vi "PXI-2510 RT Driver VI.vi"(6 "Device Clock":string, 9 "Device Inputs FIFO":refnum<k33>, 11 "Device Reference":T1 format="%.0x") -> ()   [LabVIEW 2011, in "PXI-2510 Custom Device.lvlib"]
uses:
  PXI-2510 Custom Device.lvlib
  <vilib>/NI Veristand/Custom Device API/Custom Device Item Ref.ctl
  <vilib>/NI Veristand/Custom Device API/Custom Device Channel Type.ctl
  <vilib>/Platform/TimedLoop/XDataNode/timing_clust.ctl
  <vilib>/Platform/TimedLoop/XDataNode/nitl_modes.ctl
  <vilib>/Platform/TimedLoop/XDataNode/wakeup.ctl
  <vilib>/NI Veristand/Custom Device API/Get Item Property (String).vi
  FIU Global Strings.vi
  <vilib>/Platform/TimedLoop/XDataNode/XDataNode.xnode
  <vilib>/Platform/TimedLoop/XDataNode/XDNodeRunTimeDep.lvlib
  <vilib>/NI Veristand/Custom Device API/Custom Device API.lvlib
panel:
  in  "Status Notifier":refnum<notifier>
  # "Custom Device Template\nv1.0"
  # "Use this template as a starting point for creating a custom device code module. The input controls shown here are specially named controls that the system will use to provide the device loop with data. The controls are not required for the device loop to run. For instance, if the device doesn't produce any output data, then you don't need the Device Outputs FIFO control. If you do use these controls, however, they need to have these exact names to be functional."
  # "The optional status notifier element is used to notify the RT engine of the last state of the custom device, and to indicate the device has completed execution. If this control is not used, a default No Error value is returned to the system when the device finishes execution."
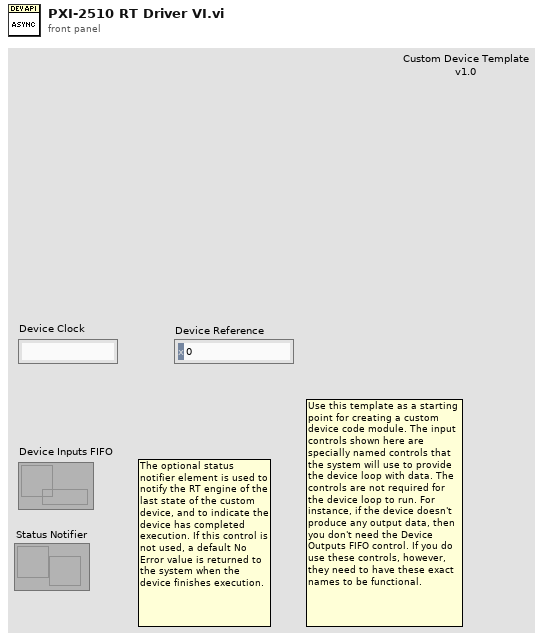
[diagram p1: front panel]
types:
  T1 = typedef "Custom Device API.lvlib/Custom Device Item Ref.ctl" = u64
  T2 = typedef "Custom Device API.lvlib/Custom Device Channel Type.ctl" = enum16{"Input", "Output"}
  T3 = typedef "Custom Device API.lvlib/Custom Device Timed Loop Priority.ctl" = enum32{"Low", "Medium", "High"}
  T4 = typedef "XDNodeRunTimeDep.lvlib/timing_clust.ctl" = cluster{"Expected End [f-1]":u64, "Actual End [f-1]":u64, "Finished Late? [f-1]":bool, "Expected End [i-1]":u64, "Actual End [i-1]":u64, "Finished Late? [i-1]":bool, "Expected Start [i]":u64, "Actual Start [i]":u64, "Expected Start [f]":u64, "Actual Start [f]":u64, "Source Name":string, "Structure Name":string, "Period":i64, "Deadline":i64, "Offset":i64, "Start":i64, "Priority":i32, "Timeout":i32, "Mode":T5, "Wakeup Reason":T6, "Error":errorcluster, "Source Type":string, "Secondary Source Type":string, "Global End Time":u64, "Global Start Time":u64, "Frame Duration":u64, "Iteration Duration":u64, "Assigned CPU":i32, "I/O Scan Engine Mode":u32}
  T5 = typedef "XDNodeRunTimeDep.lvlib/nitl_modes.ctl" = enum32{"No Change", "Process missed periods, maintain original phase", "Discard missed periods, maintain original phase", "Process missed periods, ignore original phase", "Discard missed periods, ignore original phase"}
  T6 = typedef "XDNodeRunTimeDep.lvlib/wakeup.ctl" = enum32{"Normal", "Aborted", "Asynchronous wakeup", "Timing source error", "Timed loop error", "Timeout"}
  T7 = enum16{"Default", "Fault A0 to FB A", "Fault A1 to FB A", "Fault A2 to FB A", "Fault A3 to FB A", "Fault Bus A Open"}
  T8 = enum16{"Default", "Fault B0 to FB B", "Fault B1 to FB B", "Fault B2 to FB B", "Fault B3 to FB B", "Fault Bus B Open"}
  T9 = enum16{"Default", "DUT Pass Through", "DUT Open", "DUT Pass Through and FB A", "DUT Pass Through and FB B", "DUT FB A", "DUT FB B"}
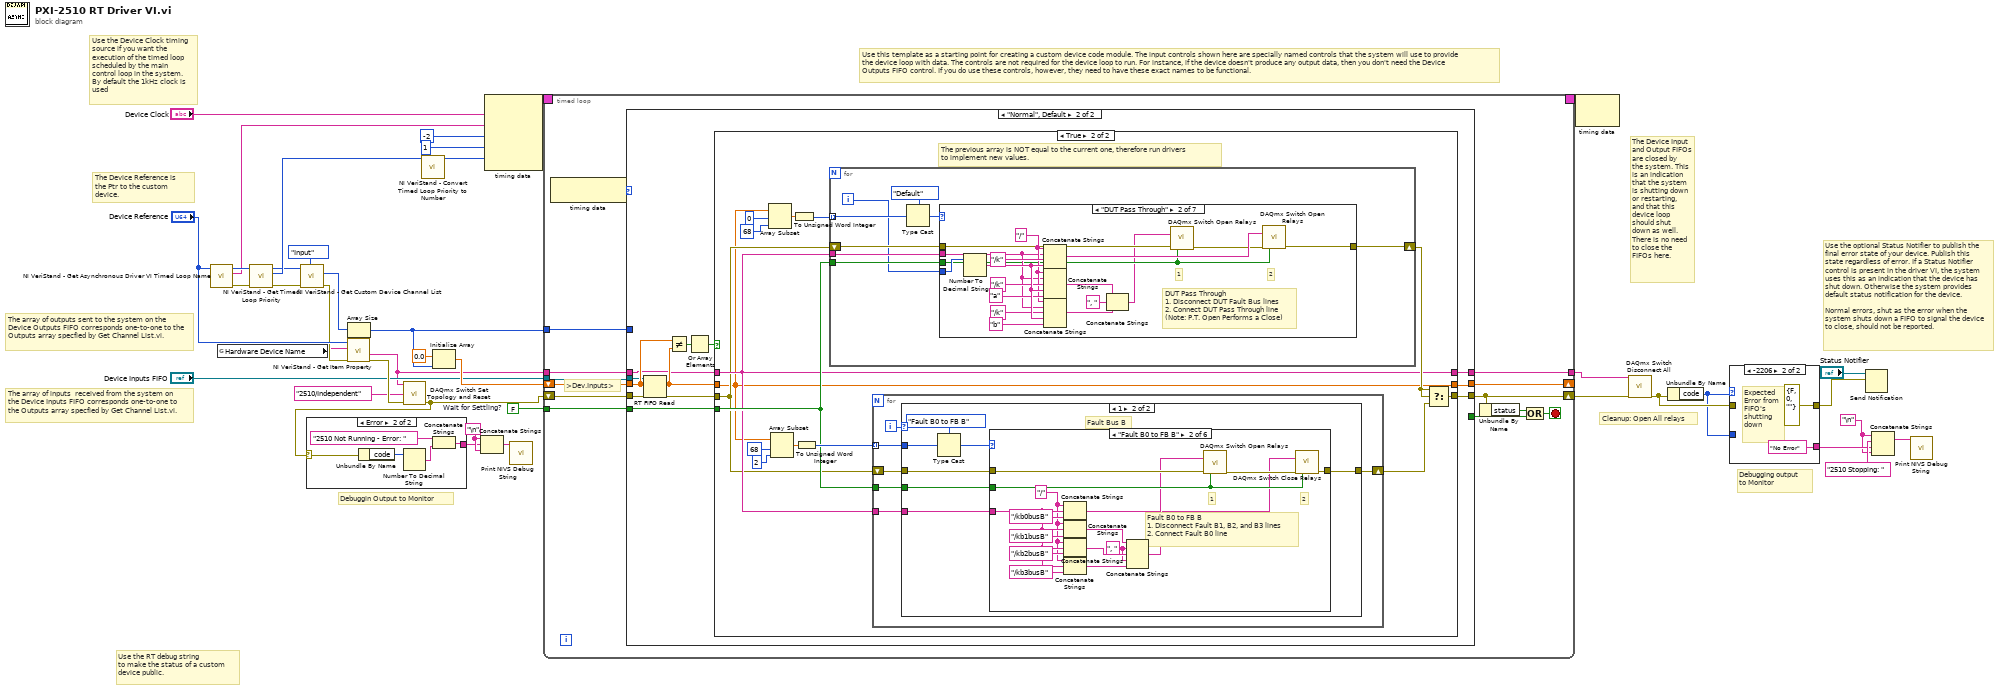
[diagram p0: block diagram]
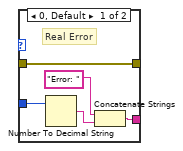
[diagram p2: hidden frame]
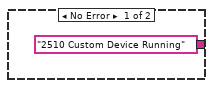
[diagram p3: hidden frame]
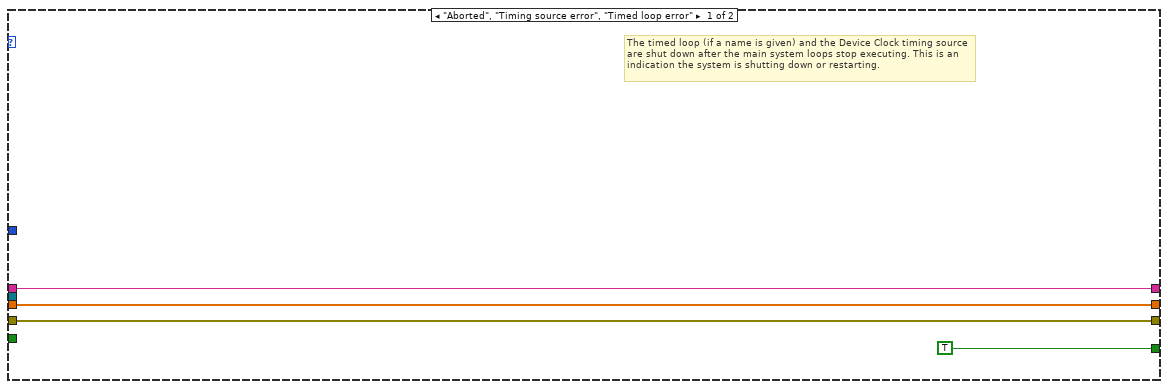
[diagram p4: hidden frame]
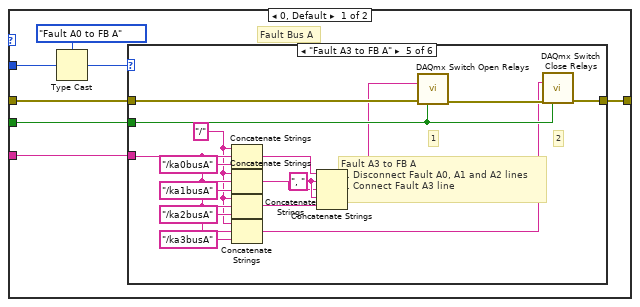
[diagram p6: hidden frame]
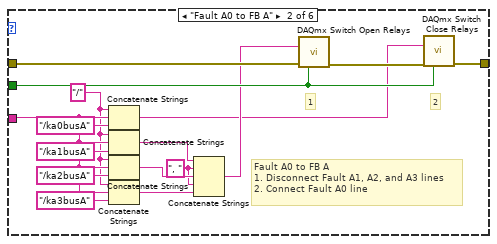
[diagram p8: hidden frame]
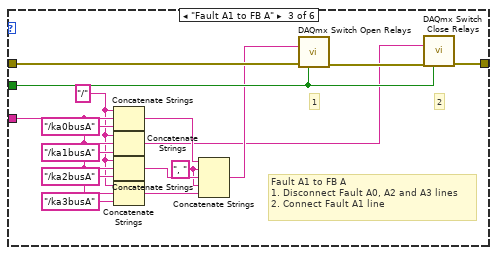
[diagram p9: hidden frame]
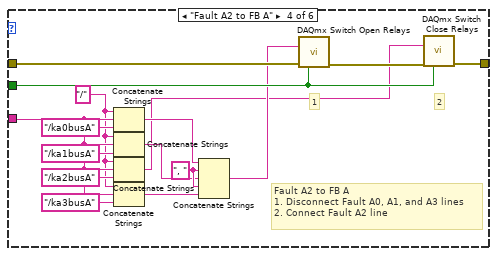
[diagram p10: hidden frame]
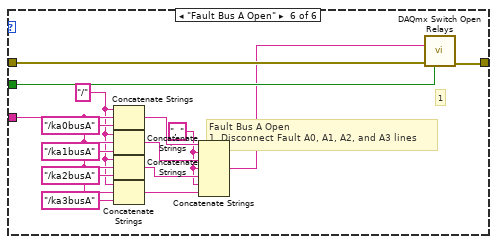
[diagram p11: hidden frame]
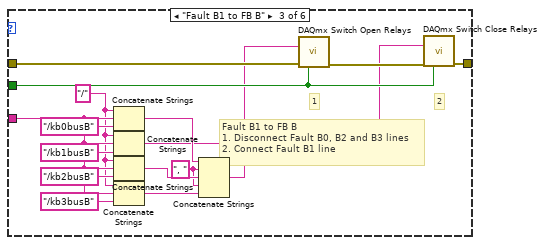
[diagram p13: hidden frame]
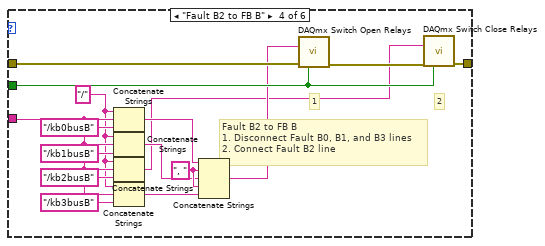
[diagram p14: hidden frame]
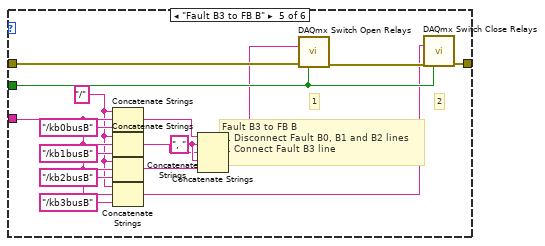
[diagram p15: hidden frame]
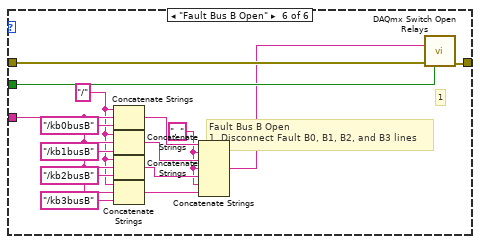
[diagram p16: hidden frame]
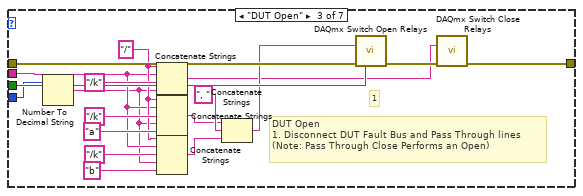
[diagram p18: hidden frame]
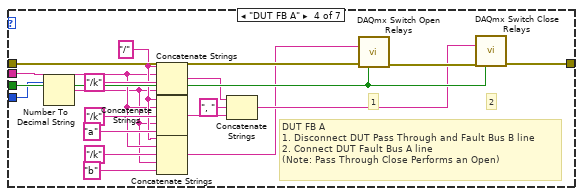
[diagram p19: hidden frame]
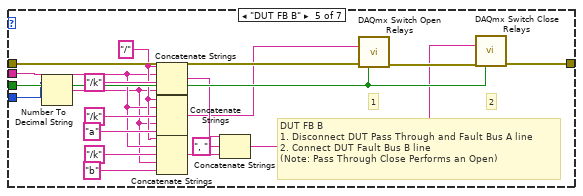
[diagram p20: hidden frame]
diagram:
  w4 = "\n"
  w14 = "\n"
  w24 = FALSE  # Wait for Settling?
  # "Debugging output\nto Monitor"
  # "Debuggin Output to Monitor"
  # "Cleanup: Open All relays"
  # "The array of inputs  received from the system on the Device Inputs FIFO corresponds one-to-one to the Outputs array specfied by Get Channel List.vi."
  # "Use the optional Status Notifier to publish the final error state of your device. Publish this state regardless of error. If a Status Notifier control is present in the driver VI, the system uses this as an indication that the device has shut down. Otherwise the system provides default status notification for the device.\n\nNormal errors, shut as the error when the system shuts down a FIFO to signal the device to close, should not be reported."
  # "Use the RT debug string\nto make the status of a custom\ndevice public."
  # "The Device Input and Output FIFOs are closed by the system. This is an indication that the system is shutting down or restarting, and that this device loop should shut down as well. There is no need to close the FIFOs here."
  # "The array of outputs sent to the system on the Device Outputs FIFO corresponds one-to-one to the Outputs array specfied by Get Channel List.vi."
  # "The Device Reference is\nthe Ptr to the custom device."
  # "Use the Device Clock timing source if you want the execution of the timed loop scheduled by the main control loop in the system. \nBy default the 1kHz clock is used"
  # "Use this template as a starting point for creating a custom device code module. The input controls shown here are specially named controls that the system will use to provide the device loop with data. The controls are not required for the device loop to run. For instance, if the device doesn't produce any output data, then you don't need the Device Outputs FIFO control. If you do use these controls, however, they need to have these exact names to be functional."
  n1 = call <vilib>:"NI VeriStand - Get Asynchronous Driver VI Timed Loop Name.vi"("Device Ref in"="Device Reference") -> ("error out"=w31:errorcluster, "Device Timed Loop Name"=w34:string, "Device Ref out"=w39:T1)  [unwired: 1 in, 7 out]
  n2 = global read "FIU Global Strings.vi" "Hardware Device Name"() -> (w19:string)
  n3 = call <vilib>:"NI VeriStand - Get Timed Loop Priority.vi"("error in (no error)"=w31, "Device Ref in"=w39) -> ("error out"=w16:errorcluster, "Priority"=w29:T3, "Device Ref out"=w17:T1)  [unwired: 7 out]
  n4 = call <vilib>:"NI VeriStand - Get Custom Device Channel List.vi"("Channel Type"=Custom_Device_Channel_Type."Input", "error in (no error)"=w16, "Device Ref in"=w17) -> ("error out"=w20:errorcluster, "Specified Channel Ref List"=w30:T1[])  [unwired: 7 out]
  n5 = call-poly <vilib>:"NI VeriStand - Get Item Property.vi"("error in (no error)"=w20, "Property Name"=w19, "Item Ref in"="Device Reference") -> ("error out"=w18:errorcluster, "Value"=w2:string)  [unwired: 5 in, 2 out]
  n6 = Array Size(array=w30) -> (size(s)=w25:i32)
  n7 = call <vilib>:"DAQmx Switch Set Topology and Reset.vi"("switch device"=w2, "topology name"="2510/Independent" ("string"), "error in"=w18) -> ("error out"=w1:errorcluster)  [unwired: 12 out]
  n8 = case shown="Error" w1 {
    selector: w1 -> [_ w41]
    tunnel: ["2510 Custom Device Running" ("String to write") w42] -> w13
    frame No Error {
    }
    frame Error {
      n9 = Unbundle By Name(w41) -> ("code"=w45:i32)
      n10 = Number To Decimal String(number=w45) -> (decimal integer string=w43:string)  [unwired: 1 in]
      n11 = Concatenate Strings("2510 Not Running - Error: " ("String to write"), w43) -> (w42:string)
    }
  }
  n12 = call <vilib>:"NI VeriStand - Convert Timed Loop Priority to Number.vi"("Priority"=w29) -> ("Numeric Priority"=w28:i32)  [unwired: 10 out]
  n13 = Initialize Array(0.0 ("element"), w25) -> (w35:dbl[])
  n14 = Concatenate Strings(w14, w13, w14) -> (w12:string)
  n15 = node-c288("Device Clock", w34, -2 ("Processor"), i64 1 ("Period"), w28) -> (w38:T4)
  n16 = call "Print NIVS Debug String.vi"("Debug String"=w12) -> ()  [unwired: 9 in, 1 out]
  n17 = timed-loop {
    timing: w38 -> [_]
    timing-out: [_] -> w37
    shift-right: [w56] -> _
    shift-left: w35 -> [w57]
    shift-right: [w54] -> w23
    shift-left: w1 -> [w58]
    tunnel: w25 -> [w50]
    tunnel: w24 -> [w49]
    tunnel: [w48] -> w22
    tunnel: "Device Inputs FIFO" -> [w47]
    tunnel: w2 -> [w46]
    stop <- w51 stop-if-true
    # ">Dev.Inputs>"
    n18 = node-c288() -> (w55:T6)  [unwired: 1 out]
    n19 = case shown="\"Normal\", Default" w55 {
      tunnel: w58 -> [w61 w69]
      tunnel: w57 -> [w62 w68]
      tunnel: [w61 w74] -> w54
      tunnel: [w62 w67] -> w56
      tunnel: [TRUE _] -> w52
      tunnel: w50 -> [_ _]
      tunnel: w49 -> [_ w73]
      tunnel: w46 -> [w59 w66]
      tunnel: [w59 w65] -> w48
      tunnel: w47 -> [_ w64]
      frame "Aborted", "Timing source error", "Timed loop error" {
        # "The timed loop (if a name is given) and the Device Clock timing source are shut down after the main system loops stop executing. This is an indication the system is shutting down or restarting."
      }
      frame "Normal", Default {
        n20 = RT FIFO Read(0:w64, 1:w68, 3:w69) -> (9:w70:dbl[], 11:w71:errorcluster)  [unwired: 1 in, 3 out]
        n21 = Not Equal?(x=w68, y=w70) -> (x != y?=w72:bool[])
        n22 = Or Array Elements(Boolean array=w72) -> (logical OR=w63:bool)
        n23 = case shown="True" w63 {
          tunnel: [w76 w92] -> w74
          tunnel: w73 -> [_ w81]
          tunnel: w71 -> [w76 w79]
          tunnel: w70 -> [w77 w78]
          tunnel: [w77 w78] -> w67
          tunnel: w66 -> [w75 w80]
          tunnel: [w75 w80] -> w65
          frame False {
            # "The previous array is equal to the current one, therefore no values have changed and there is no reason\nto run the driver calls again."
          }
          frame True {
            # "The previous array is NOT equal to the current one, therefore run drivers\nto implement new values."
            n24 = Array Subset(array=w78, index=0, length=68) -> (w85:dbl[])
            n25 = Array Subset(array=w78, index=68, length=2) -> (w84:dbl[])
            n26 = To Unsigned Word Integer(number=w85) -> (unsigned 16bit integer=w83:u16[])
            n27 = To Unsigned Word Integer(number=w84) -> (unsigned 16bit integer=w82:u16[])
            n28 = for {
              tunnel: w83 -> [w280] mode=indexing
              tunnel: w81 -> [w278]
              shift-right: [w277] -> w91
              shift-left: w79 -> [w279]
              tunnel: w80 -> [w276]
              i -> [w275]
              n29 = Type Cast(type=T9."Default", x=w280) -> (*(type *) &x=w273:T9)
              n30 = case shown="\"DUT Pass Through\"" w273 {
                tunnel: w279 -> [w281 w298 w317 w334 w352 w371 w388]
                tunnel: [w281 w299 w301 w335 w353 w357 w389] -> w277
                tunnel: w278 -> [_ w284 w316 w332 w350 w370 w386]
                tunnel: w275 -> [_ w290 w305 w330 w348 w368 w384]
                tunnel: w276 -> [_ w285 w308 w323 w341 w361 w377]
                frame Default {
                }
                frame "DUT Pass Through" {
                  w286 = "/" ("string")
                  # "2"
                  # "1"
                  # "DUT Pass Through\n1. Disconnect DUT Fault Bus lines\n2. Connect DUT Pass Through line\n(Note: P.T. Open Performs a Close)"
                  n31 = Number To Decimal String(number=w290) -> (decimal integer string=w296:string)  [unwired: 1 in]
                  n32 = Concatenate Strings(w286, w285, "/k", w296) -> (w289:string)
                  n33 = Concatenate Strings(w286, w285, "/k", w296, "a") -> (w288:string)
                  n34 = Concatenate Strings(w286, w285, "/k", w296, "b") -> (w287:string)
                  n35 = Concatenate Strings(w288, ", " ("string"), w287) -> (w283:string)
                  n36 = call <vilib>:"DAQmx Switch Open Relays.vi"("relays"=w283, "error in"=w298, "wait for settling"=w284) -> ("error out"=w282:errorcluster)  [unwired: 12 out]
                  n37 = call <vilib>:"DAQmx Switch Open Relays.vi"("relays"=w289, "error in"=w282, "wait for settling"=w284) -> ("error out"=w299:errorcluster)  [unwired: 12 in]
                }
                frame "DUT Open" {
                  w309 = "/" ("string")
                  # "1"
                  # "DUT Open\n1. Disconnect DUT Fault Bus and Pass Through lines\n(Note: Pass Through Close Performs an Open)"
                  n38 = Number To Decimal String(number=w305) -> (decimal integer string=w304:string)  [unwired: 1 in]
                  n39 = Concatenate Strings(w309, w308, "/k", w304) -> (w300:string)
                  n40 = Concatenate Strings(w309, w308, "/k", w304, "a") -> (w307:string)
                  n41 = Concatenate Strings(w309, w308, "/k", w304, "b") -> (w306:string)
                  n42 = Concatenate Strings(w307, ", " ("string"), w306) -> (w303:string)
                  n43 = call <vilib>:"DAQmx Switch Open Relays.vi"("relays"=w303, "error in"=w317, "wait for settling"=w316) -> ("error out"=w302:errorcluster)  [unwired: 12 out]
                  n44 = call <vilib>:"DAQmx Switch Close Relays.vi"("relays"=w300, "error in"=w302) -> ("error out"=w301:errorcluster)  [unwired: 13 in]
                }
                frame "DUT FB A" {
                  w324 = "/" ("string")
                  # "2"
                  # "1"
                  # "DUT FB A\n1. Disconnect DUT Pass Through and Fault Bus B line\n2. Connect DUT Fault Bus A line\n(Note: Pass Through Close Performs an Open)"
                  n45 = Number To Decimal String(number=w330) -> (decimal integer string=w322:string)  [unwired: 1 in]
                  n46 = Concatenate Strings(w324, w323, "/k", w322) -> (w321:string)
                  n47 = Concatenate Strings(w324, w323, "/k", w322, "a") -> (w320:string)
                  n48 = Concatenate Strings(w324, w323, "/k", w322, "b") -> (w318:string)
                  n49 = Concatenate Strings(w321, ", " ("string"), w320) -> (w319:string)
                  n50 = call <vilib>:"DAQmx Switch Open Relays.vi"("relays"=w318, "error in"=w334, "wait for settling"=w332) -> ("error out"=w333:errorcluster)  [unwired: 12 out]
                  n51 = call <vilib>:"DAQmx Switch Close Relays.vi"("relays"=w319, "error in"=w333, "wait for settling"=w332) -> ("error out"=w335:errorcluster)  [unwired: 12 out]
                }
                frame "DUT FB B" {
                  w342 = "/" ("string")
                  # "2"
                  # "1"
                  # "DUT FB B\n1. Disconnect DUT Pass Through and Fault Bus A line\n2. Connect DUT Fault Bus B line\n(Note: Pass Through Close Performs an Open)"
                  n52 = Number To Decimal String(number=w348) -> (decimal integer string=w340:string)  [unwired: 1 in]
                  n53 = Concatenate Strings(w342, w341, "/k", w340) -> (w339:string)
                  n54 = Concatenate Strings(w342, w341, "/k", w340, "a") -> (w336:string)
                  n55 = Concatenate Strings(w342, w341, "/k", w340, "b") -> (w338:string)
                  n56 = Concatenate Strings(w339, ", " ("string"), w338) -> (w337:string)
                  n57 = call <vilib>:"DAQmx Switch Open Relays.vi"("relays"=w336, "error in"=w352, "wait for settling"=w350) -> ("error out"=w351:errorcluster)  [unwired: 12 out]
                  n58 = call <vilib>:"DAQmx Switch Close Relays.vi"("relays"=w337, "error in"=w351, "wait for settling"=w350) -> ("error out"=w353:errorcluster)  [unwired: 12 out]
                }
                frame "DUT Pass Through and FB A" {
                  w362 = "/" ("string")
                  # "2"
                  # "1"
                  # "DUT Pass Through and FB A\n1. Disconnect DUT Fault Bus B line\n2. Connect DUT Pass Through and Fault Bus A line\n(Note: Pass Through Open Performs a Close)"
                  n59 = Number To Decimal String(number=w368) -> (decimal integer string=w360:string)  [unwired: 1 in]
                  n60 = Concatenate Strings(w362, w361, "/k", w360) -> (w359:string)
                  n61 = Concatenate Strings(w362, w361, "/k", w360, "a") -> (w354:string)
                  n62 = Concatenate Strings(w362, w361, "/k", w360, "b") -> (w356:string)
                  n63 = Concatenate Strings(w359, ", " ("string"), w356) -> (w355:string)
                  n64 = call <vilib>:"DAQmx Switch Open Relays.vi"("relays"=w355, "error in"=w371, "wait for settling"=w370) -> ("error out"=w358:errorcluster)  [unwired: 12 out]
                  n65 = call <vilib>:"DAQmx Switch Close Relays.vi"("relays"=w354, "error in"=w358, "wait for settling"=w370) -> ("error out"=w357:errorcluster)  [unwired: 12 out]
                }
                frame "DUT Pass Through and FB B" {
                  w378 = "/" ("string")
                  # "2"
                  # "1"
                  # "DUT Pass Through and FB B\n1. Disconnect DUT Fault Bus A line\n2. Connect DUT Pass Through and Fault Bus B line\n(Note: Pass Through Open Performs a Close)"
                  n66 = Number To Decimal String(number=w384) -> (decimal integer string=w376:string)  [unwired: 1 in]
                  n67 = Concatenate Strings(w378, w377, "/k", w376) -> (w375:string)
                  n68 = Concatenate Strings(w378, w377, "/k", w376, "a") -> (w374:string)
                  n69 = Concatenate Strings(w378, w377, "/k", w376, "b") -> (w372:string)
                  n70 = Concatenate Strings(w375, ", " ("string"), w374) -> (w373:string)
                  n71 = call <vilib>:"DAQmx Switch Open Relays.vi"("relays"=w373, "error in"=w388, "wait for settling"=w386) -> ("error out"=w387:errorcluster)  [unwired: 12 out]
                  n72 = call <vilib>:"DAQmx Switch Close Relays.vi"("relays"=w372, "error in"=w387, "wait for settling"=w386) -> ("error out"=w389:errorcluster)  [unwired: 12 out]
                }
              }
            }
            n73 = for {
              tunnel: w82 -> [w97] mode=indexing
              tunnel: w81 -> [w95]
              shift-right: [w94] -> w90
              shift-left: w79 -> [w96]
              tunnel: w80 -> [w93]
              i -> [w98]
              n74 = case shown="1" w98 {
                tunnel: w97 -> [w105 w192]
                tunnel: w96 -> [w103 w191]
                tunnel: w95 -> [w102 w190]
                tunnel: [w101 w189] -> w94
                tunnel: w93 -> [w99 w187]
                frame 0, Default {
                  # "Fault Bus A"
                  n75 = Type Cast(type=T7."Fault A0 to FB A" ("Fault Channel Operations"), x=w105) -> (*(type *) &x=w100:T7)
                  n76 = case shown="\"Fault A3 to FB A\"" w100 {
                    tunnel: w103 -> [w106 w121 w137 w153 w169 w185]
                    tunnel: [w106 w122 w138 w154 w170 w184] -> w101
                    tunnel: w102 -> [_ w119 w135 w151 w167 w183]
                    tunnel: w99 -> [_ w112 w127 w144 w161 w175]
                    frame Default {
                    }
                    frame "Fault A0 to FB A" {
                      w107 = "/" ("string")
                      w111 = ", " ("string")
                      # "2"
                      # "1"
                      # "Fault A0 to FB A\n1. Disconnect Fault A1, A2, and A3 lines\n2. Connect Fault A0 line"
                      n77 = Concatenate Strings(w107, w112, "/ka0busA") -> (w108:string)
                      n78 = Concatenate Strings(w107, w112, "/ka1busA") -> (w115:string)
                      n79 = Concatenate Strings(w107, w112, "/ka2busA") -> (w114:string)
                      n80 = Concatenate Strings(w107, w112, "/ka3busA") -> (w110:string)
                      n81 = Concatenate Strings(w115, w111, w114, w111, w110) -> (w109:string)
                      n82 = call <vilib>:"DAQmx Switch Open Relays.vi"("relays"=w109, "error in"=w121, "wait for settling"=w119) -> ("error out"=w120:errorcluster)  [unwired: 12 out]
                      n83 = call <vilib>:"DAQmx Switch Close Relays.vi"("relays"=w108, "error in"=w120, "wait for settling"=w119) -> ("error out"=w122:errorcluster)  [unwired: 12 out]
                    }
                    frame "Fault A1 to FB A" {
                      w123 = "/" ("string")
                      w129 = ", " ("string")
                      # "2"
                      # "1"
                      # "Fault A1 to FB A\n1. Disconnect Fault A0, A2 and A3 lines\n2. Connect Fault A1 line"
                      n84 = Concatenate Strings(w123, w127, "/ka0busA") -> (w126:string)
                      n85 = Concatenate Strings(w123, w127, "/ka1busA") -> (w124:string)
                      n86 = Concatenate Strings(w123, w127, "/ka2busA") -> (w131:string)
                      n87 = Concatenate Strings(w123, w127, "/ka3busA") -> (w128:string)
                      n88 = Concatenate Strings(w126, w129, w131, w129, w128) -> (w125:string)
                      n89 = call <vilib>:"DAQmx Switch Open Relays.vi"("relays"=w125, "error in"=w137, "wait for settling"=w135) -> ("error out"=w136:errorcluster)  [unwired: 12 out]
                      n90 = call <vilib>:"DAQmx Switch Close Relays.vi"("relays"=w124, "error in"=w136, "wait for settling"=w135) -> ("error out"=w138:errorcluster)  [unwired: 12 out]
                    }
                    frame "Fault A2 to FB A" {
                      w139 = "/" ("string")
                      w146 = ", " ("string")
                      # "2"
                      # "1"
                      # "Fault A2 to FB A\n1. Disconnect Fault A0, A1, and A3 lines\n2. Connect Fault A2 line"
                      n91 = Concatenate Strings(w139, w144, "/ka0busA") -> (w142:string)
                      n92 = Concatenate Strings(w139, w144, "/ka1busA") -> (w143:string)
                      n93 = Concatenate Strings(w139, w144, "/ka2busA") -> (w140:string)
                      n94 = Concatenate Strings(w139, w144, "/ka3busA") -> (w145:string)
                      n95 = Concatenate Strings(w142, w146, w143, w146, w145) -> (w141:string)
                      n96 = call <vilib>:"DAQmx Switch Open Relays.vi"("relays"=w141, "error in"=w153, "wait for settling"=w151) -> ("error out"=w152:errorcluster)  [unwired: 12 out]
                      n97 = call <vilib>:"DAQmx Switch Close Relays.vi"("relays"=w140, "error in"=w152, "wait for settling"=w151) -> ("error out"=w154:errorcluster)  [unwired: 12 out]
                    }
                    frame "Fault A3 to FB A" {
                      w155 = "/" ("string")
                      w162 = ", " ("string")
                      # "2"
                      # "1"
                      # "Fault A3 to FB A\n1. Disconnect Fault A0, A1 and A2 lines\n2. Connect Fault A3 line"
                      n98 = Concatenate Strings(w155, w161, "/ka0busA") -> (w160:string)
                      n99 = Concatenate Strings(w155, w161, "/ka1busA") -> (w159:string)
                      n100 = Concatenate Strings(w155, w161, "/ka2busA") -> (w158:string)
                      n101 = Concatenate Strings(w155, w161, "/ka3busA") -> (w156:string)
                      n102 = Concatenate Strings(w160, w162, w159, w162, w158) -> (w157:string)
                      n103 = call <vilib>:"DAQmx Switch Open Relays.vi"("relays"=w157, "error in"=w169, "wait for settling"=w167) -> ("error out"=w168:errorcluster)  [unwired: 12 out]
                      n104 = call <vilib>:"DAQmx Switch Close Relays.vi"("relays"=w156, "error in"=w168, "wait for settling"=w167) -> ("error out"=w170:errorcluster)  [unwired: 12 out]
                    }
                    frame "Fault Bus A Open" {
                      w171 = "/" ("string")
                      w173 = ", " ("string")
                      # "1"
                      # "Fault Bus A Open\n1. Disconnect Fault A0, A1, A2, and A3 lines"
                      n105 = Concatenate Strings(w171, w175, "/ka0busA") -> (w174:string)
                      n106 = Concatenate Strings(w171, w175, "/ka1busA") -> (w179:string)
                      n107 = Concatenate Strings(w171, w175, "/ka2busA") -> (w178:string)
                      n108 = Concatenate Strings(w171, w175, "/ka3busA") -> (w176:string)
                      n109 = Concatenate Strings(w174, w173, w179, w173, w178, w173, w176) -> (w172:string)
                      n110 = call <vilib>:"DAQmx Switch Open Relays.vi"("relays"=w172, "error in"=w185, "wait for settling"=w183) -> ("error out"=w184:errorcluster)  [unwired: 12 out]
                    }
                  }
                }
                frame 1 {
                  # "Fault Bus B"
                  n111 = Type Cast(type=T8."Fault B0 to FB B" ("Fault Channel Operations"), x=w192) -> (*(type *) &x=w188:T8)
                  n112 = case shown="\"Fault B0 to FB B\"" w188 {
                    tunnel: w191 -> [w193 w208 w224 w240 w256 w272]
                    tunnel: [w193 w209 w225 w241 w257 w271] -> w189
                    tunnel: w190 -> [_ w206 w222 w238 w254 w270]
                    tunnel: w187 -> [_ w199 w214 w231 w248 w262]
                    frame Default {
                    }
                    frame "Fault B0 to FB B" {
                      w194 = "/" ("string")
                      w198 = ", " ("string")
                      # "2"
                      # "1"
                      # "Fault B0 to FB B\n1. Disconnect Fault B1, B2, and B3 lines\n2. Connect Fault B0 line"
                      n113 = Concatenate Strings(w194, w199, "/kb0busB") -> (w195:string)
                      n114 = Concatenate Strings(w194, w199, "/kb1busB") -> (w202:string)
                      n115 = Concatenate Strings(w194, w199, "/kb2busB") -> (w201:string)
                      n116 = Concatenate Strings(w194, w199, "/kb3busB") -> (w197:string)
                      n117 = Concatenate Strings(w202, w198, w201, w198, w197) -> (w196:string)
                      n118 = call <vilib>:"DAQmx Switch Open Relays.vi"("relays"=w196, "error in"=w208, "wait for settling"=w206) -> ("error out"=w207:errorcluster)  [unwired: 12 out]
                      n119 = call <vilib>:"DAQmx Switch Close Relays.vi"("relays"=w195, "error in"=w207, "wait for settling"=w206) -> ("error out"=w209:errorcluster)  [unwired: 12 out]
                    }
                    frame "Fault B1 to FB B" {
                      w210 = "/" ("string")
                      w216 = ", " ("string")
                      # "2"
                      # "1"
                      # "Fault B1 to FB B\n1. Disconnect Fault B0, B2 and B3 lines\n2. Connect Fault B1 line"
                      n120 = Concatenate Strings(w210, w214, "/kb0busB") -> (w213:string)
                      n121 = Concatenate Strings(w210, w214, "/kb1busB") -> (w211:string)
                      n122 = Concatenate Strings(w210, w214, "/kb2busB") -> (w218:string)
                      n123 = Concatenate Strings(w210, w214, "/kb3busB") -> (w215:string)
                      n124 = Concatenate Strings(w213, w216, w218, w216, w215) -> (w212:string)
                      n125 = call <vilib>:"DAQmx Switch Open Relays.vi"("relays"=w212, "error in"=w224, "wait for settling"=w222) -> ("error out"=w223:errorcluster)  [unwired: 12 out]
                      n126 = call <vilib>:"DAQmx Switch Close Relays.vi"("relays"=w211, "error in"=w223, "wait for settling"=w222) -> ("error out"=w225:errorcluster)  [unwired: 12 out]
                    }
                    frame "Fault B2 to FB B" {
                      w226 = "/" ("string")
                      w233 = ", " ("string")
                      # "2"
                      # "1"
                      # "Fault B2 to FB B\n1. Disconnect Fault B0, B1, and B3 lines\n2. Connect Fault B2 line"
                      n127 = Concatenate Strings(w226, w231, "/kb0busB") -> (w229:string)
                      n128 = Concatenate Strings(w226, w231, "/kb1busB") -> (w230:string)
                      n129 = Concatenate Strings(w226, w231, "/kb2busB") -> (w227:string)
                      n130 = Concatenate Strings(w226, w231, "/kb3busB") -> (w232:string)
                      n131 = Concatenate Strings(w229, w233, w230, w233, w232) -> (w228:string)
                      n132 = call <vilib>:"DAQmx Switch Open Relays.vi"("relays"=w228, "error in"=w240, "wait for settling"=w238) -> ("error out"=w239:errorcluster)  [unwired: 12 out]
                      n133 = call <vilib>:"DAQmx Switch Close Relays.vi"("relays"=w227, "error in"=w239, "wait for settling"=w238) -> ("error out"=w241:errorcluster)  [unwired: 12 out]
                    }
                    frame "Fault B3 to FB B" {
                      w242 = "/" ("string")
                      w249 = ", " ("string")
                      # "2"
                      # "1"
                      # "Fault B3 to FB B\n1. Disconnect Fault B0, B1 and B2 lines\n2. Connect Fault B3 line"
                      n134 = Concatenate Strings(w242, w248, "/kb0busB") -> (w247:string)
                      n135 = Concatenate Strings(w242, w248, "/kb1busB") -> (w246:string)
                      n136 = Concatenate Strings(w242, w248, "/kb2busB") -> (w245:string)
                      n137 = Concatenate Strings(w242, w248, "/kb3busB") -> (w243:string)
                      n138 = Concatenate Strings(w247, w249, w246, w249, w245) -> (w244:string)
                      n139 = call <vilib>:"DAQmx Switch Open Relays.vi"("relays"=w244, "error in"=w256, "wait for settling"=w254) -> ("error out"=w255:errorcluster)  [unwired: 12 out]
                      n140 = call <vilib>:"DAQmx Switch Close Relays.vi"("relays"=w243, "error in"=w255, "wait for settling"=w254) -> ("error out"=w257:errorcluster)  [unwired: 12 out]
                    }
                    frame "Fault Bus B Open" {
                      w258 = "/" ("string")
                      w260 = ", " ("string")
                      # "1"
                      # "Fault Bus B Open\n1. Disconnect Fault B0, B1, B2, and B3 lines"
                      n141 = Concatenate Strings(w258, w262, "/kb0busB") -> (w261:string)
                      n142 = Concatenate Strings(w258, w262, "/kb1busB") -> (w266:string)
                      n143 = Concatenate Strings(w258, w262, "/kb2busB") -> (w265:string)
                      n144 = Concatenate Strings(w258, w262, "/kb3busB") -> (w263:string)
                      n145 = Concatenate Strings(w261, w260, w266, w260, w265, w260, w263) -> (w259:string)
                      n146 = call <vilib>:"DAQmx Switch Open Relays.vi"("relays"=w259, "error in"=w272, "wait for settling"=w270) -> ("error out"=w271:errorcluster)  [unwired: 12 out]
                    }
                  }
                }
              }
            }
            n147 = Select(t=w91, s=w91, f=w90) -> (s? t:f=w92:errorcluster)
          }
        }
      }
    }
    n148 = Unbundle By Name(w54) -> ("status"=w53:bool)
    n149 = Compound Arithmetic op=OR(w53, w52) -> (w51:bool)
  }
  n150 = node-c288(w37) -> ()  [unwired: 1 out]
  n151 = call <vilib>:"DAQmx Switch Disconnect All.vi"("switch device"=w22, "error in"=w23) -> ("error out"=w9:errorcluster)  [unwired: 1 in, 12 out]
  n152 = Unbundle By Name(w9) -> ("code"=w3:i32)
  n153 = case shown="-2206" w3 {
    tunnel: w9 -> [w397 _]
    tunnel: [w397 errorcluster {"status"=FALSE, "code"=0, "source"=""} ("error out")] -> w8
    tunnel: [w393 "No Error" ("string")] -> w5
    tunnel: w3 -> [w396 _]
    frame 0, Default {
      # "Real Error"
      n154 = Number To Decimal String(number=w396) -> (decimal integer string=w394:string)  [unwired: 1 in]
      n155 = Concatenate Strings("Error: " ("string"), w394) -> (w393:string)
    }
    frame -2206 {
      # "Expected\nError from\nFIFO's \nshutting\ndown"
    }
  }
  n156 = Send Notification(notification=w8, notifier="Status Notifier") -> ()  [unwired: 1 in, 2 out]
  n157 = Concatenate Strings "Concatenate Strings"(w4, "2510 Stopping: " ("string"), w5, w4) -> (w7:string)
  n158 = call "Print NIVS Debug String.vi"("Debug String"=w7) -> ()  [unwired: 9 in, 1 out]
